vi "PH_Periodic_Sequencer.constructor.vi"(0 "name":string, 2 "data in":string, 5 "error in(no error)":errorcluster) -> (14 "i ref out":refnum<vi>, 16 "data out":string, 19 "error out":errorcluster)   [LabVIEW 2014, in "PH_Periodic_Sequencer.lvlib"]
doc: "The Sequencer controlles the PHELIX shot procedure.\n\nThis class is part of the PHELIX user layer.\n\nauthor: Stefan Götte, GSI\n\nLicense Agreement for this software:\n\nCopyright (C)\nGesellschaft für Schwerionenforschung, GSI\nPlanckstr. 1\n64291 Darmstadt\nGermany\n\nContact: D.Beck@gsi.de \n\nThis program is free software; you can redistribute it and/or modify it under the terms of the \nGNU General Public License as published by the Free Software Foundation; either version 2 of \nthe license, or (at your option) any later version.\n\nThis program is distributed in the hope that it will be useful, but WITHOUT ANY WARRANTY; \nwithout even the implied warranty of MERCHANTABILITY or FITNESS FOR A PARTICULAR PURPOSE. See the GNU General License for more details (http://www.gnu.org).\n\nGesellschaft für Schwerionenforschung, GSI\nPlanckstr. 1, 64291 Darmstadt, Germany\nFor all questions and ideas contact: M.Richter@gsi.de, H.Brand@gsi.de or D.Beck@gsi.de.\nLast update: 16-JUN-2004"
uses:
  PH_Periodic_Sequencer.lvlib
  CSCore/CSObj/CSObj.lvlib
  PH_Class/PH_Class.lvlib
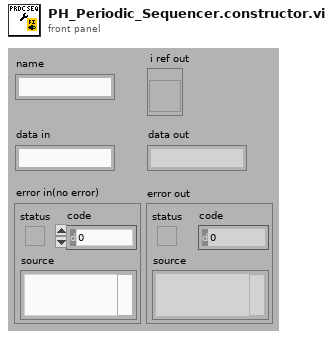
[diagram p1: front panel]
types:
  T1 = enum16{"SetAttribute", "GetAttribute", "CreateAttribute", "DestroyAttribute", "DestroyAllAtributes"}
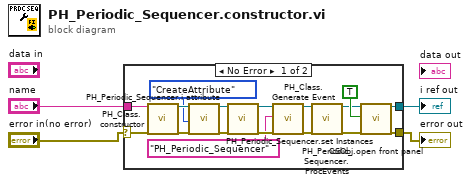
[diagram p0: block diagram]
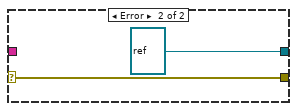
[diagram p2: hidden frame]
diagram:
  n1 = case shown="No Error" "error in(no error)" {
    selector: "error in(no error)" -> [w16 w23]
    tunnel: "name" -> [w21 _]
    tunnel: [w14 w23] -> w3
    tunnel: [w15 refnum<vi> refnum ("i ref out")] -> w2
    frame No Error {
      n2 = call "PH_Class.constructor.vi"("name"=w21, "error in"=w16) -> ("i ref out"=w19:refnum<vi>, "error out"=w20:errorcluster)  [unwired: 15 in, 1 out]
      n3 = call "PH_Periodic_Sequencer.i attribute.vi"("VI Refnum"=w19, "Action"=T1."CreateAttribute", "error in (no error)"=w20) -> ("VI Refnum out"=w10:refnum<vi>, "error out"=w11:errorcluster)  [unwired: 14 in, 1 out]
      n4 = call "PH_Periodic_Sequencer.set Instances.vi"("i ref in"=w10, "error in (no error)"=w11) -> ("i ref out"=w7:refnum<vi>, "error out"=w6:errorcluster)  [unwired: 16 in]
      n5 = call "PH_Class.Generate Event.vi"("i ref in"=w7, "Class"="PH_Periodic_Sequencer", "error in (no error)"=w6) -> ("i ref out"=w13:refnum<vi>, "error out"=w12:errorcluster)  [unwired: 15 in]
      n6 = call "PH_Periodic_Sequencer.ProcEvents.vi"("i ref in"=w13, "error in (no error)"=w12) -> ("i ref out"=w9:refnum<vi>, "error out"=w8:errorcluster)  [unwired: 16 in]
      n7 = call "CSObj.open front panel.vi"("i ref in"=w9, "frontPanelOpen"=TRUE ("front panel open"), "error in (no error)"=w8) -> ("i ref out"=w15:refnum<vi>, "error out"=w14:errorcluster)  [unwired: 15 in]
    }
    frame Error {
    }
  }
  "i ref out" <- w2
  "error out" <- w3
